vi "dll.midi_file_get_track_info.vi"(8 "error in (no error)":errorcluster, 10 "Track Index":i32, 11 "midi file in":refnum<class "midi file.lvclass">) -> (0 "error out":errorcluster, 2 "Track Info":T1, 3 "midi file out":refnum<class "midi file.lvclass">)   [LabVIEW 2020, in "midi file.lvclass"]
uses:
  midi file.lvclass
  track info.ctl
  midi file.lvclass/midi file.ctl
  shared/midi shared.lvlib
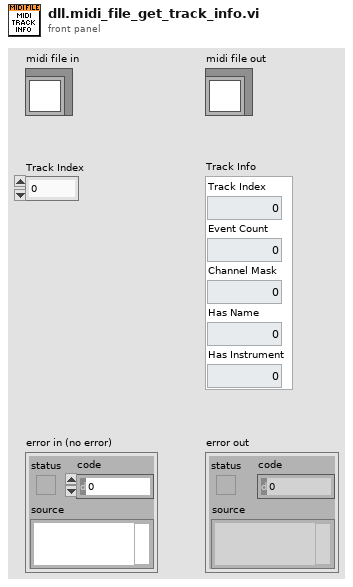
[diagram p1: front panel]
types:
  T1 = typedef "midi file.lvclass/track info.ctl" = cluster{"Track Index":i32, "Event Count":i32, "Channel Mask":i32, "Has Name":i32, "Has Instrument":i32}
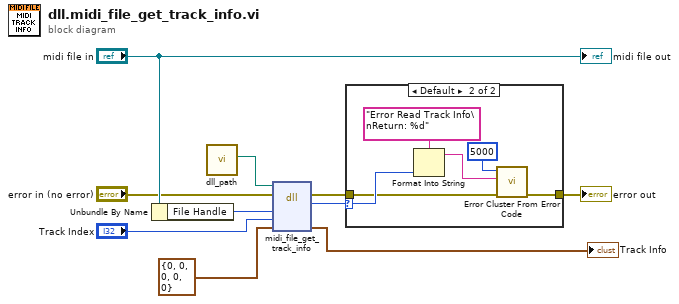
[diagram p0: block diagram]
diagram:
  n1 = Unbundle By Name("midi file in") -> ("File Handle"=w6:i32)
  n2 = call "dll_path.vi"() -> ("dll"=w10:path)  [unwired: 11 in]
  n3 = dll-call lib="C:/code/LabVIEW-MIDI-XPLAT/dist/TomMIDIllan_*.*" fn="midi_file_get_track_info"(path in=w10, error in="error in (no error)", "File Handle"=w6, "Track Index"="Track Index", "Track Info Cluster"=T1 {"Track Index"=0, "Event Count"=0, "Channel Mask"=0, "Has Name"=0, "Has Instrument"=0} ("Track Info")) -> (error out=w9:errorcluster, "Error code"=w8:i32, "Track Info Cluster"=→"Track Info":T1)  [unwired: 3 in, 1 out]
  n4 = case shown="Default" w8 {
    selector: w8 -> [_ w14]
    tunnel: w9 -> [w11 w13]
    tunnel: [w11 w12] -> w4
    frame 0.. {
    }
    frame Default {
      n5 = Format Into String(format string="Error Read Track Info\nReturn: %d", w14) -> (resulting string=w15:string)  [unwired: 2 in, 1 out]
      n6 = call <vilib>:"Error Cluster From Error Code.vi"("error in (no error)"=w13, "error message (\"\")"=w15, "error code (0)"=5000) -> ("error out"=w12:errorcluster)  [unwired: 6 in]
    }
  }
  "error out" <- w4
  "midi file out" <- "midi file in"
